vi "Main.vi"(11 "Module Admin":refnum<class "Delacor_lib_QMH_Cloneable Module Admin.lvclass">) -> ()   [LabVIEW 2025, in "USB IO.lvlib"]
doc: "This template is based off of the Queued Message Handler design pattern and the Queued Message Handler project template that ships with LabVIEW.\n\nThe main difference is that the queue is private to this module and communication between modules is performed via Broadcast and Request events.\n\nRequest events are wrapped in public API methods and are handled in the Event Handling Loop (EHL) of this VI. Any module can register for Broadcast events sent by this module. The EHL generates messages based on user interface actions.\n\nThe Message Handling Loop (MHL) processes messages generated by the EHL, or by other messages. The messages are string values, so new messages can be added easily to the Message Cases case structure in the MHL. Each message cluster can also provide an optional value for Message Data, which is a variant that can be converted to whatever message-specific data is required.\n_____\nBased on DQMH Dev Tools: Project Template 7.1.2.1547."
uses:
  USB IO.lvlib
  <vilib>/Delacor/Delacor QMH/Libraries/Message Queue_class/Delacor_lib_QMH_Message Queue.lvclass
  Module Data--cluster.ctl
  <vilib>/Utility/miscctls.llb/LVPointTypeDef.ctl
  <vilib>/Delacor/Delacor QMH/Libraries/Message Queue_class/Delacor_lib_QMH_Enqueue Message (Single).vi
  Stop Argument--cluster.ctl
  <vilib>/Delacor/Delacor QMH/Libraries/Cloneable Module Admin_class/Delacor_lib_QMH_Cloneable Module Admin.lvclass
  Display Lines (Reply Payload)--cluster.ctl
  Display Lines Argument--cluster.ctl
  Classes/USB IO generic/USB IO.lvclass
  select child (Reply Payload)--cluster.ctl
  Classes/Hardware Selection.ctl
  select child Argument--cluster.ctl
  Classes/Arduino Uno/Arduino Uno.lvclass
  Classes/USB-6000/USB-6000.lvclass
  read config (Reply Payload)--cluster.ctl
  read config Argument--cluster.ctl
  init device (Reply Payload)--cluster.ctl
  init device Argument--cluster.ctl
  stop device (Reply Payload)--cluster.ctl
  stop device Argument--cluster.ctl
  Controls/Numeric Voltage.ctl
  analog read (Reply Payload)--cluster.ctl
  analog read Argument--cluster.ctl
  digital write (Reply Payload)--cluster.ctl
  digital write Argument--cluster.ctl
  C:/Users/Tyson.Grover/Desktop/Repositories/torque-test-station/Libraries/USB IO/Classes/USB IO generic/USB IO.lvclass
  C:/Users/Tyson.Grover/Desktop/Repositories/torque-test-station/Libraries/USB IO/Classes/USB-6000/USB-6000.lvclass
  C:/Users/Tyson.Grover/Desktop/Repositories/torque-test-station/Libraries/USB IO/Classes/Arduino Uno/Arduino Uno.lvclass
panel:
  out "error out":errorcluster
  out "Status":string
  in  "Simulate EHL Error":bool
  in  "Simulate MHL Error":bool
  # "Other processes communicate with this Module via its Public API (wrappers for its Request Events).\n\nThis Module communicates with other processes via its Broadcast Events.\nAny process that wants to receive these messages can register for this module's Broadcast events."
  # "This template is for the DQMH framework. See the block diagram for more information on how to use this template."
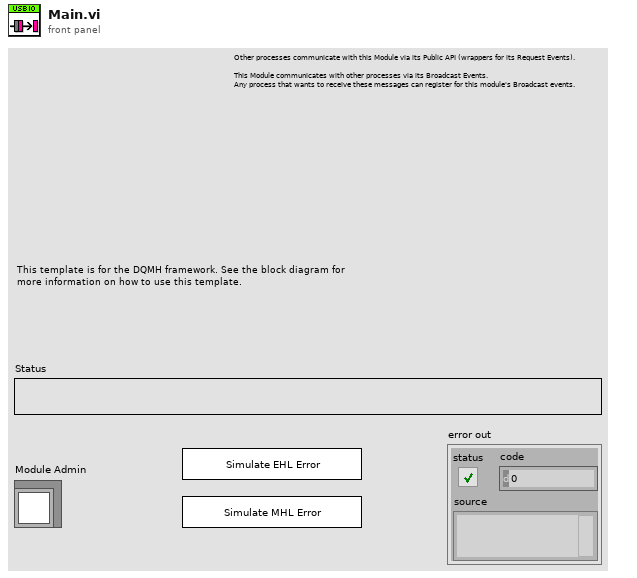
[diagram p1: front panel]
types:
  T1 = typedef "USB IO.lvlib/Request Events--cluster.ctl" = cluster{"Stop Module":refnum<user-event>, "Show Panel":refnum<user-event>, "Hide Panel":refnum<user-event>, "Show Diagram":refnum<user-event>, "Get Module Execution Status":refnum<user-event>, "Display Lines":refnum<user-event>, "select child":refnum<user-event>, "read config":refnum<user-event>, "init":refnum<user-event>, "init device":refnum<user-event>, "stop device":refnum<user-event>, "analog read":refnum<user-event>, "digital write":refnum<user-event>}
  T2 = typedef "USB IO.lvlib/Module Data--cluster.ctl" = cluster{"Status":string, "USB IO.lvlib:USB IO.lvclass":refnum<class "USB IO.lvclass">}
  T3 = enum32{"invalid lock state", "Not Locked", "Locked (No Password)", "Password-protected"}
  T4 = typedef "USB IO.lvlib/Stop Argument--cluster.ctl" = cluster{"Module ID":i32, "Origin":string, "Exit via Stop Module Req?":bool, "Wait for Module to stop?":bool}
  T5 = typedef "USB IO.lvlib/Display Lines Argument--cluster.ctl" = cluster{"Module ID":i32, "Wait Notifier":refnum<notifier>, "wait for reply":bool}
  T6 = typedef "USB IO.lvlib/select child Argument--cluster.ctl" = cluster{"Module ID":i32, "Hardware":T7, "Wait Notifier":refnum<notifier>, "wait for reply":bool}
  T7 = typedef "Hardware Selection.ctl" = enum16{"Simulation", "USB-6000", "USB-6001", "Arduino Uno"}
  T8 = typedef "USB IO.lvlib/read config Argument--cluster.ctl" = cluster{"Module ID":i32, "Path":path, "Wait Notifier":refnum<notifier>, "wait for reply":bool}
  T9 = typedef "USB IO.lvlib/init device Argument--cluster.ctl" = cluster{"Module ID":i32, "Variant":variant, "Wait Notifier":refnum<notifier>, "wait for reply":bool}
  T10 = typedef "USB IO.lvlib/stop device Argument--cluster.ctl" = cluster{"Module ID":i32, "Wait Notifier":refnum<notifier>, "wait for reply":bool}
  T11 = typedef "USB IO.lvlib/analog read Argument--cluster.ctl" = cluster{"Module ID":i32, "Line":string, "Wait Notifier":refnum<notifier>, "wait for reply":bool}
  T12 = typedef "USB IO.lvlib/digital write Argument--cluster.ctl" = cluster{"Module ID":i32, "Line":string, "On/Off":bool, "Wait Notifier":refnum<notifier>, "wait for reply":bool}
  T13 = typedef "LVPointTypeDef.ctl" = cluster{"Horizontal":i16, "Vertical":i16}
  T14 = enum32{"Invalid", "Standard", "Closed", "Hidden", "Minimized", "Maximized"}
  T15 = typedef "USB IO.lvlib/Display Lines (Reply Payload)--cluster.ctl" = cluster{"Module ID":i32, "Lines":string[], "Values":i32[], "error":errorcluster}
  T16 = typedef "USB IO.lvlib/select child (Reply Payload)--cluster.ctl" = cluster{"Module ID":i32, "error":errorcluster}
  T17 = typedef "USB IO.lvlib/read config (Reply Payload)--cluster.ctl" = cluster{"Module ID":i32, "error":errorcluster}
  T18 = typedef "USB IO.lvlib/init device (Reply Payload)--cluster.ctl" = cluster{"Module ID":i32, "error":errorcluster}
  T19 = typedef "USB IO.lvlib/stop device (Reply Payload)--cluster.ctl" = cluster{"Module ID":i32, "error":errorcluster}
  T20 = typedef "USB IO.lvlib/analog read (Reply Payload)--cluster.ctl" = cluster{"Module ID":i32, "Voltage":T21, "error":errorcluster}
  T21 = typedef "Numeric Voltage.ctl" = dbl
  T22 = typedef "USB IO.lvlib/digital write (Reply Payload)--cluster.ctl" = cluster{"Module ID":i32, "error":errorcluster}
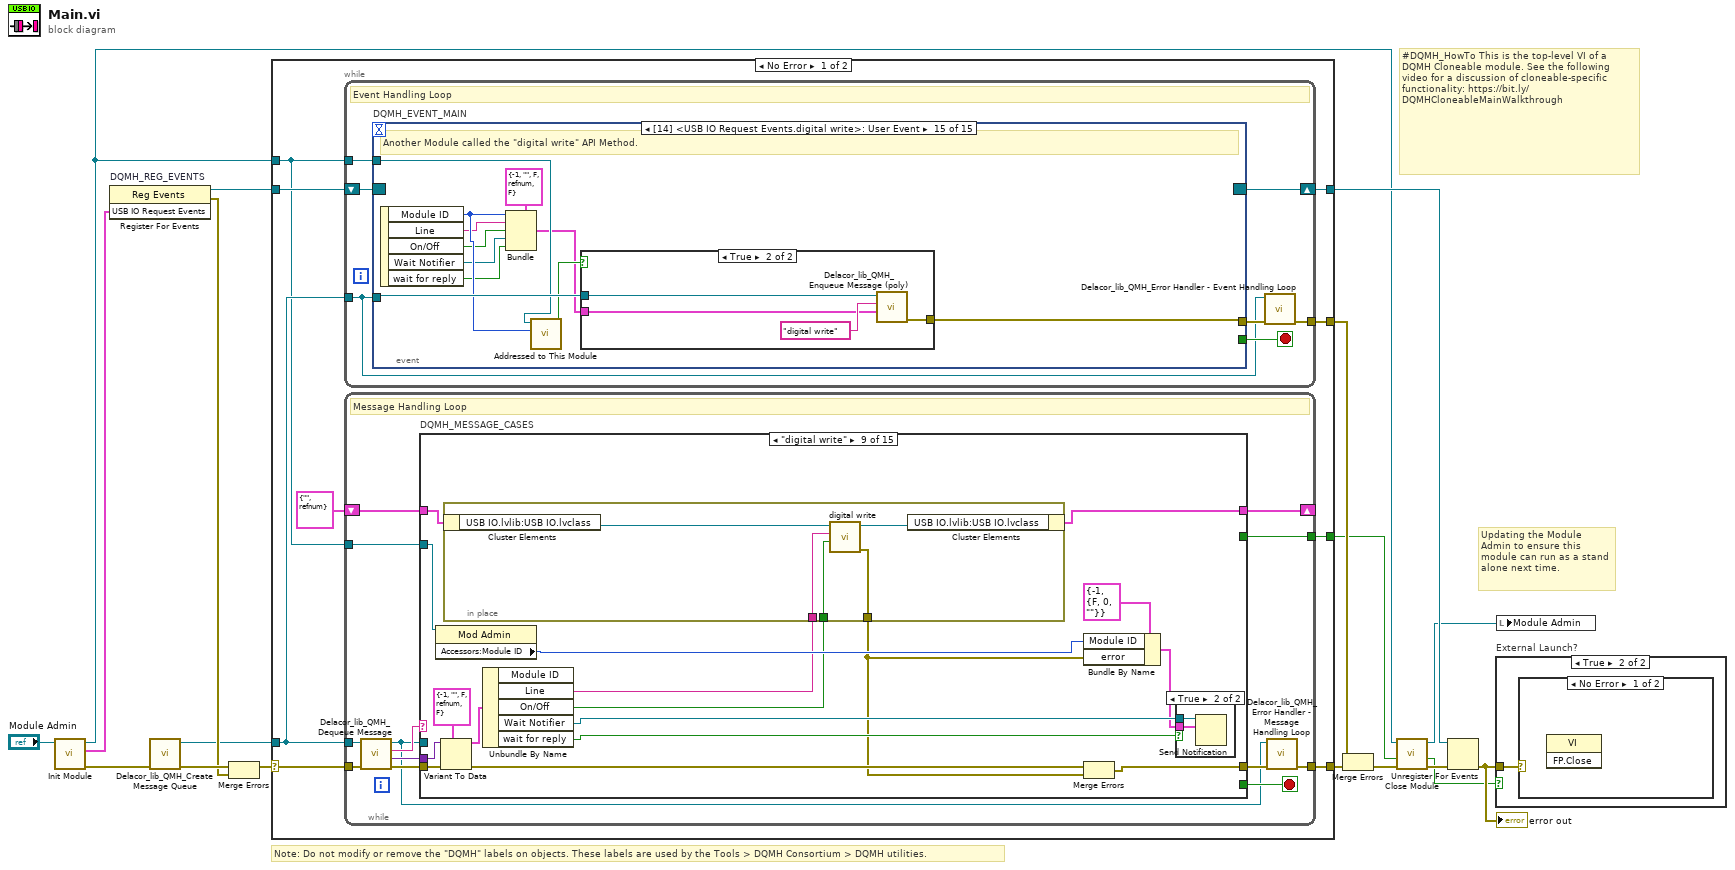
[diagram p0: block diagram]
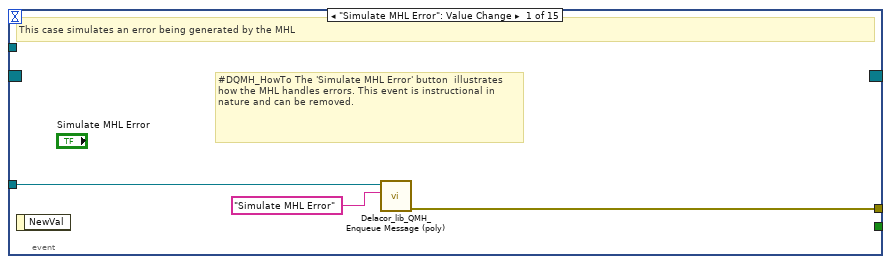
[diagram p2: hidden frame]
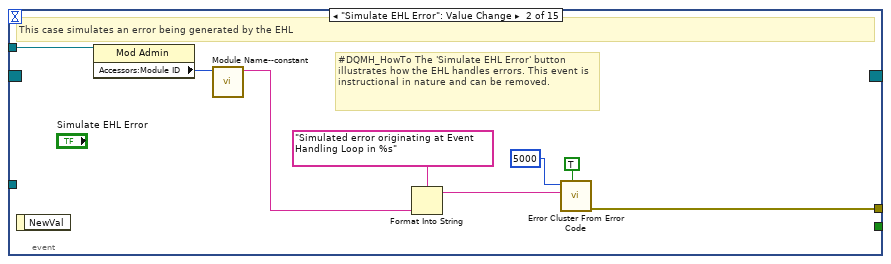
[diagram p3: hidden frame]
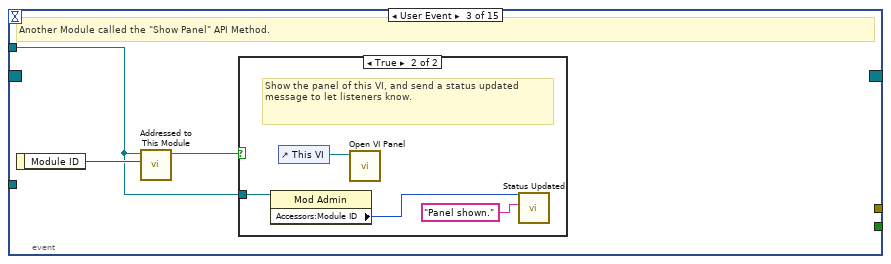
[diagram p4: hidden frame]
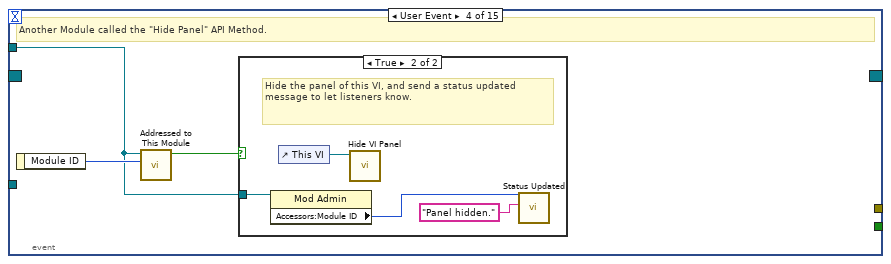
[diagram p6: hidden frame]
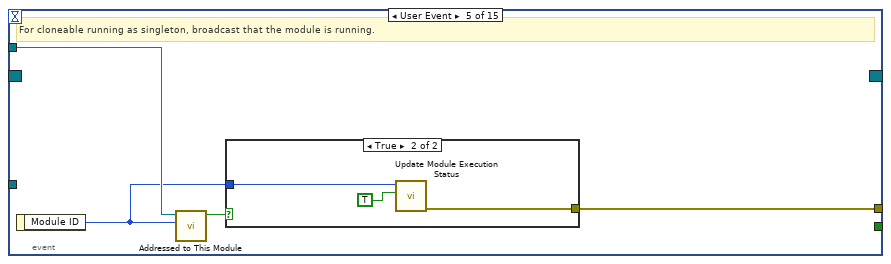
[diagram p8: hidden frame]
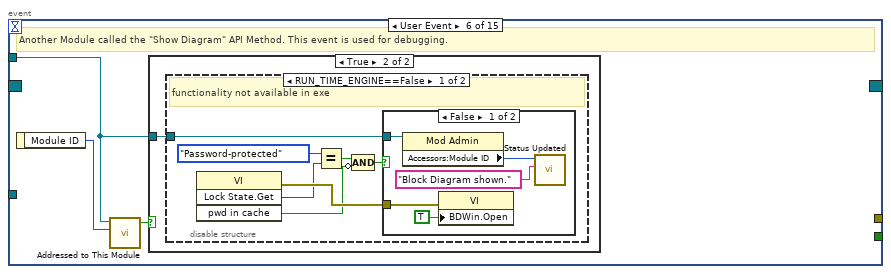
[diagram p10: hidden frame]
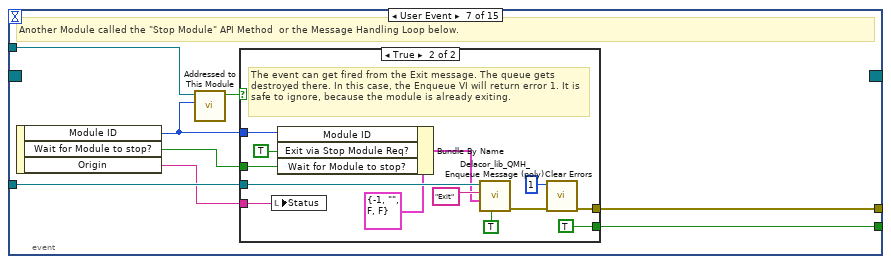
[diagram p14: hidden frame]
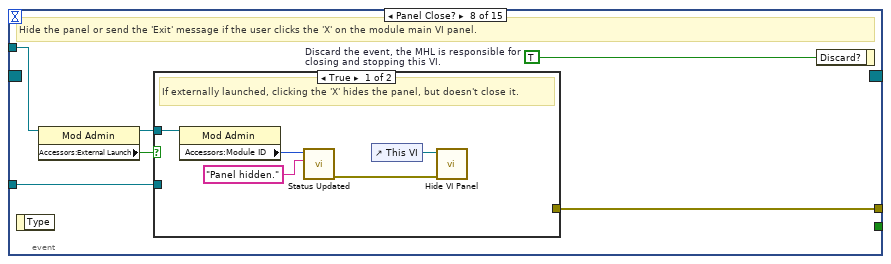
[diagram p16: hidden frame]
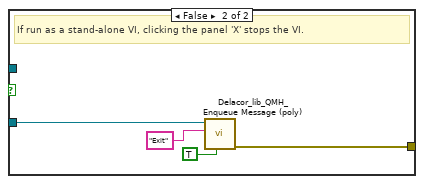
[diagram p17: hidden frame]
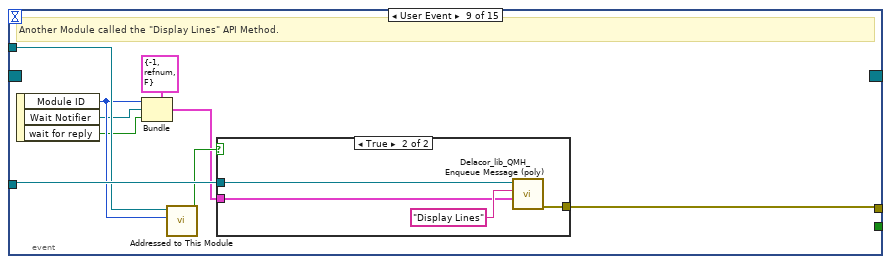
[diagram p18: hidden frame]
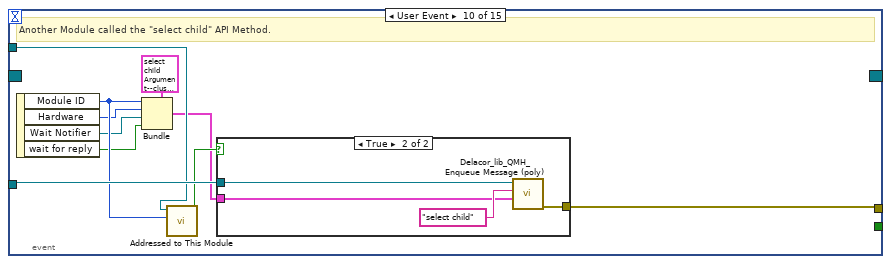
[diagram p20: hidden frame]
diagram:
  # "#DQMH_HowTo This is the top-level VI of a DQMH Cloneable module. See the following video for a discussion of cloneable-specific functionality: https://bit.ly/DQMHCloneableMainWalkthrough"
  # "Note: Do not modify or remove the \"DQMH\" labels on objects. These labels are used by the Tools > DQMH Consortium > DQMH utilities."
  # "Updating the Module Admin to ensure this module can run as a stand alone next time."
  n1 = call "Init Module.vi"("Cloneable Module Admin in"="Module Admin") -> ("error out"=w15:errorcluster, "USB IO Request Events"=w7:T1, "Cloneable Module Admin out"=w4:refnum<class "Delacor_lib_QMH_Cloneable Module Admin.lvclass">)  [unwired: 8 in]
  n2 = register-events "DQMH_REG_EVENTS"(w7) -> (reference out=w8:refnum<event-registration>, error out=w10:errorcluster)  [unwired: 2 in]
  n3 = call <vilib>:"Delacor_lib_QMH_Create Message Queue.vi"("error in"=w15) -> ("error out"=w12:errorcluster, "Message Queue"=w6:refnum<class "Delacor_lib_QMH_Message Queue.lvclass">)  [unwired: 9 in]
  n4 = Merge Errors(w12, w10) -> (w11:errorcluster)
  n5 = case shown="No Error" w11 {
    selector: w11 -> [w25 w482]
    tunnel: [w27 w481] -> w16
    tunnel: [w24 w480] -> w9
    tunnel: w8 -> [w22 w480]
    tunnel: w6 -> [w21 w473]
    tunnel: [w26 _] -> w17
    tunnel: w4 -> [w20 w476]
    tunnel: [w19 _] -> w2
    frame No Error {
      n6 = while {
        tunnel: w21 -> [w28]
        shift-right: [w31] -> w24
        shift-left: w22 -> [w32]
        tunnel: [w33] -> w26
        tunnel: w20 -> [w29]
        stop <- w30 stop-if-true
        # "Event Handling Loop"
        n7 = event "DQMH_EVENT_MAIN" shown="[14] <USB IO Request Events.digital write>: User Event" {
          selector: w32 -> [_ _ _ _ _ _ _ _ _ _ _ _ _ _ _]
          dyn-events: [_ _ _ _ _ _ _ _ _ _ _ _ _ _ _] -> w31
          timeout: _ -> [_ _ _ _ _ _ _ _ _ _ _ _ _ _ _]
          tunnel: [_ _ _ _ _ _ w86 _ _ _ _ _ _ _ _] -> w30
          tunnel: w28 -> [w36 _ _ _ _ _ w89 w106 w127 w141 w155 w169 w182 w196 w211]
          tunnel: [w37 w45 _ _ w63 _ w90 w109 w119 w132 w146 w160 w174 w187 w201] -> w34
          tunnel: w29 -> [_ w44 w46 w53 w61 w67 w88 w107 w125 w139 w153 w167 w180 w194 w209]
          event "Simulate MHL Error": Value Change {
            # "#DQMH_HowTo The 'Simulate MHL Error' button  illustrates how the MHL handles errors. This event is instructional in nature and can be removed."
            # "This case simulates an error being generated by the MHL"
            n8 = event-data() -> ()  [unwired: 1 in, 1 out]
            n9 = call-poly <vilib>:"Delacor_lib_QMH_Enqueue Message (poly).vi"("Message"="Simulate MHL Error", "Message Queue in"=w36) -> ("error out"=w37:errorcluster)  [unwired: 8 in, 1 out]
          }
          event "Simulate EHL Error": Value Change {
            # "#DQMH_HowTo The 'Simulate EHL Error' button  illustrates how the EHL handles errors. This event is instructional in nature and can be removed."
            # "This case simulates an error being generated by the EHL"
            n10 = event-data() -> ()  [unwired: 1 in, 1 out]
            n11 = property on="Property Node" class="Mod Admin"(reference=w44) -> ("Accessors:Module ID"=w43:i32)  [unwired: 1 in, 2 out]
            n12 = call "Module Name--constant.vi"("Module ID"=w43) -> ("Module Name"=w38:string)  [unwired: 10 in]
            n13 = Format Into String(format string="Simulated error originating at Event Handling Loop in %s", w38) -> (resulting string=w41:string)  [unwired: 2 in, 1 out]
            n14 = call <vilib>:"Error Cluster From Error Code.vi"("show call chain? (False)"=TRUE, "error message (\"\")"=w41, "error code (0)"=5000) -> ("error out"=w45:errorcluster)  [unwired: 6 in]
          }
          event User Event {
            # "Another Module called the \"Show Panel\" API Method."
            n15 = event-data() -> ("Module ID"=w47:i32)  [unwired: 1 in]
            n16 = call "Addressed to This Module.vi"("Module ID from Argument"=w47, "Module Admin"=w46) -> ("Addressed to this instance?"=w48:bool)  [unwired: 8 in, 1 out]
            n17 = case shown="True" w48 {
              tunnel: w46 -> [_ w50]
              frame False {
              }
              frame True {
                # "Show the panel of this VI, and send a status updated message to let listeners know."
                n18 = property on="Property Node" class="Mod Admin"(reference=w50) -> ("Accessors:Module ID"=w49:i32)  [unwired: 1 in, 2 out]
                n19 = control-ref of="This VI"() -> (w52:refnum<vi>)
                n20 = call "Open VI Panel.vi"("VI"=w52) -> ()  [unwired: 10 in, 1 out]
                n21 = call "Status Updated.vi"("Status"="Panel shown." ("format string"), "Module ID"=w49) -> ()  [unwired: 9 in, 1 out]
              }
            }
          }
          event User Event {
            # "Another Module called the \"Hide Panel\" API Method."
            n22 = event-data() -> ("Module ID"=w54:i32)  [unwired: 1 in]
            n23 = call "Addressed to This Module.vi"("Module ID from Argument"=w54, "Module Admin"=w53) -> ("Addressed to this instance?"=w55:bool)  [unwired: 8 in, 1 out]
            n24 = case shown="True" w55 {
              tunnel: w53 -> [_ w57]
              frame False {
              }
              frame True {
                # "Hide the panel of this VI, and send a status updated message to let listeners know."
                n25 = property on="Property Node" class="Mod Admin"(reference=w57) -> ("Accessors:Module ID"=w56:i32)  [unwired: 1 in, 2 out]
                n26 = control-ref of="This VI"() -> (w59:refnum<vi>)
                n27 = call "Hide VI Panel.vi"("VI"=w59) -> ()  [unwired: 10 in, 1 out]
                n28 = call "Status Updated.vi"("Status"="Panel hidden." ("format string"), "Module ID"=w56) -> ()  [unwired: 9 in, 1 out]
              }
            }
          }
          event User Event {
            # "For cloneable running as singleton, broadcast that the module is running."
            n29 = event-data() -> ("Module ID"=w60:i32)  [unwired: 1 in]
            n30 = call "Addressed to This Module.vi"("Module ID from Argument"=w60, "Module Admin"=w61) -> ("Addressed to this instance?"=w62:bool)  [unwired: 8 in, 1 out]
            n31 = case shown="True" w62 {
              tunnel: [_ w66] -> w63
              tunnel: w60 -> [_ w65]
              frame False {
              }
              frame True {
                n32 = call "Update Module Execution Status.vi"("Running?"=TRUE, "Module ID"=w65) -> ("error out"=w66:errorcluster)  [unwired: 9 in]
              }
            }
          }
          event User Event {
            # "Another Module called the \"Show Diagram\" API Method. This event is used for debugging."
            n33 = event-data() -> ("Module ID"=w68:i32)  [unwired: 1 in]
            n34 = call "Addressed to This Module.vi"("Module ID from Argument"=w68, "Module Admin"=w67) -> ("Addressed to this instance?"=w69:bool)  [unwired: 8 in, 1 out]
            n35 = case shown="True" w69 {
              tunnel: w67 -> [_ w70]
              frame False {
              }
              frame True {
                n36 = disable-structure shown="RUN_TIME_ENGINE==False" {
                  disable-tunnel: w70 -> [w71 _]
                  frame condition #0 (active) {
                    # "functionality not available in exe"
                    n37 = invoke on="Invoke Node" class="VI" method="Lock State.Get"() -> (error out=w77:errorcluster, "Get Lock State"=w76:T3, "pwd in cache"=w73:bool)  [unwired: 4 in, 1 out]
                    n38 = Equal?(x=T3."Password-protected", y=w76) -> (x = y?=w74:bool)
                    n39 = Compound Arithmetic op=AND(w74, invert w73) -> (w72:bool)
                    n40 = case shown="False" w72 {
                      tunnel: w77 -> [w82 _]
                      tunnel: w71 -> [w79 _]
                      frame False {
                        n41 = property on="Property Node" class="Mod Admin"(reference=w79) -> ("Accessors:Module ID"=w78:i32)  [unwired: 1 in, 2 out]
                        n42 = property on="Property Node" class="VI"(error in=w82, "BDWin.Open"=TRUE ("Block Diagram Window:Open")) -> ()  [unwired: 1 in, 2 out]
                        n43 = call "Status Updated.vi"("Status"="Block Diagram shown." ("format string"), "Module ID"=w78) -> ()  [unwired: 9 in, 1 out]
                      }
                      frame True {
                        # "Password-protected VI, and the password is not in the cache. Do not show the diagram."
                      }
                    }
                  }
                  frame condition #1 {
                  }
                }
              }
            }
          }
          event User Event {
            # "Another Module called the \"Stop Module\" API Method  or the Message Handling Loop below."
            n44 = event-data() -> ("Module ID"=w84:i32, "Wait for Module to stop?"=w85:bool, "Origin"=w83:string)  [unwired: 1 in]
            n45 = call "Addressed to This Module.vi"("Module ID from Argument"=w84, "Module Admin"=w88) -> ("Addressed to this instance?"=w87:bool)  [unwired: 8 in, 1 out]
            n46 = case shown="True" w87 {
              tunnel: [_ w102] -> w90
              tunnel: w89 -> [_ w98]
              tunnel: [_ TRUE] -> w86
              tunnel: w85 -> [_ w93]
              tunnel: w84 -> [_ w95]
              tunnel: w83 -> [_ w91]
              frame False {
              }
              frame True {
                # "The event can get fired from the Exit message. The queue gets destroyed there. In this case, the Enqueue VI will return error 1. It is safe to ignore, because the module is already exiting."
                n47 = local write "Status"(w91) -> ()
                n48 = Bundle By Name(cluster=T4 {"Module ID"=-1, "Origin"="", "Exit via Stop Module Req?"=FALSE, "Wait for Module to stop?"=FALSE} ("Stop Argument"), "Module ID"=w95, "Exit via Stop Module Req?"=TRUE, "Wait for Module to stop?"=w93) -> (w92:T4)
                n49 = call-poly <vilib>:"Delacor_lib_QMH_Enqueue Message (poly).vi"("Priority Message? (F)"=TRUE, "Message Data"=w92, "Message"="Exit", "Message Queue in"=w98) -> ("error out"=w103:errorcluster)  [unwired: 6 in, 1 out]
                n50 = call <vilib>:"Clear Errors.vi"("error in (no error)"=w103, "specific error code to clear (0: all)"=1) -> ("error out"=w102:errorcluster)  [unwired: 4 in, 1 out]
              }
            }
          }
          event Panel Close? {
            w108 = TRUE  # Discard the event, the MHL is responsible for closing and stopping this VI.
            # "Hide the panel or send the 'Exit' message if the user clicks the 'X' on the module main VI panel."
            n51 = event-data() -> ()  [unwired: 1 in, 1 out]
            n52 = property on="Property Node" class="Mod Admin"(reference=w107) -> (reference out=w104:refnum<class "Delacor_lib_QMH_Cloneable Module Admin.lvclass">, "Accessors:External Launch"=w105:bool)  [unwired: 1 in, 1 out]
            n53 = case shown="True" w105 {
              tunnel: w106 -> [_ w117]
              tunnel: [_ w118] -> w109
              tunnel: w104 -> [w112 _]
              frame True {
                # "If externally launched, clicking the 'X' hides the panel, but doesn't close it."
                n54 = property on="Property Node" class="Mod Admin"(reference=w112) -> ("Accessors:Module ID"=w111:i32)  [unwired: 1 in, 2 out]
                n55 = call "Status Updated.vi"("Status"="Panel hidden." ("format string"), "Module ID"=w111) -> ("error out"=w110:errorcluster)  [unwired: 9 in]
                n56 = control-ref of="This VI"() -> (w114:refnum<vi>)
                n57 = call "Hide VI Panel.vi"("error in"=w110, "VI"=w114) -> ()  [unwired: 9 in, 1 out]
              }
              frame False {
                # "If run as a stand-alone VI, clicking the panel 'X' stops the VI."
                n58 = call-poly <vilib>:"Delacor_lib_QMH_Enqueue Message (poly).vi"("Priority Message? (F)"=TRUE, "Message"="Exit", "Message Queue in"=w117) -> ("error out"=w118:errorcluster)  [unwired: 7 in, 1 out]
              }
            }
            n59 = event-data ("Event Filter Node")("Discard?"=w108) -> ()  [unwired: 1 in, 1 out]
          }
          event User Event {
            # "Another Module called the \"Display Lines\" API Method."
            n60 = event-data() -> ("Module ID"=w122:i32, "Wait Notifier"=w121:refnum<notifier>, "wait for reply"=w120:bool)  [unwired: 1 in]
            n61 = Bundle(cluster=T5 {"Module ID"=-1, "Wait Notifier"=refnum, "wait for reply"=FALSE} ("Display Lines Argument"), "Module ID"=w122, "Wait Notifier"=w121, "wait for reply"=w120) -> (w123:T5)
            n62 = call "Addressed to This Module.vi"("Module ID from Argument"=w122, "Module Admin"=w125) -> ("Addressed to this instance?"=w126:bool)  [unwired: 8 in, 1 out]
            n63 = case shown="True" w126 {
              tunnel: w127 -> [_ w131]
              tunnel: w123 -> [_ w129]
              tunnel: [_ w128] -> w119
              frame False {
              }
              frame True {
                n64 = call-poly <vilib>:"Delacor_lib_QMH_Enqueue Message (poly).vi"("Message Data"=w129, "Message"="Display Lines", "Message Queue in"=w131) -> ("error out"=w128:errorcluster)  [unwired: 7 in, 1 out]
              }
            }
          }
          event User Event {
            # "Another Module called the \"select child\" API Method."
            n65 = event-data() -> ("Module ID"=w136:i32, "Hardware"=w135:T7, "Wait Notifier"=w134:refnum<notifier>, "wait for reply"=w133:bool)  [unwired: 1 in]
            n66 = Bundle(cluster=T6 {"Module ID"=-1, "Hardware"=enum."USB-6000", "Wait Notifier"=refnum, "wait for reply"=FALSE} ("select child Argument"), "Module ID"=w136, "Hardware"=w135, "Wait Notifier"=w134, "wait for reply"=w133) -> (w137:T6)
            n67 = call "Addressed to This Module.vi"("Module ID from Argument"=w136, "Module Admin"=w139) -> ("Addressed to this instance?"=w140:bool)  [unwired: 8 in, 1 out]
            n68 = case shown="True" w140 {
              tunnel: w141 -> [_ w145]
              tunnel: w137 -> [_ w143]
              tunnel: [_ w142] -> w132
              frame False {
              }
              frame True {
                n69 = call-poly <vilib>:"Delacor_lib_QMH_Enqueue Message (poly).vi"("Message Data"=w143, "Message"="select child", "Message Queue in"=w145) -> ("error out"=w142:errorcluster)  [unwired: 7 in, 1 out]
              }
            }
          }
          event User Event {
            # "Another Module called the \"read config\" API Method."
            n70 = event-data() -> ("Module ID"=w150:i32, "Path"=w149:path, "Wait Notifier"=w148:refnum<notifier>, "wait for reply"=w147:bool)  [unwired: 1 in]
            n71 = Bundle(cluster=T8 {"Module ID"=-1, "Path"=path "", "Wait Notifier"=refnum, "wait for reply"=FALSE} ("read config Argument"), "Module ID"=w150, "Path"=w149, "Wait Notifier"=w148, "wait for reply"=w147) -> (w151:T8)
            n72 = call "Addressed to This Module.vi"("Module ID from Argument"=w150, "Module Admin"=w153) -> ("Addressed to this instance?"=w154:bool)  [unwired: 8 in, 1 out]
            n73 = case shown="True" w154 {
              tunnel: w155 -> [_ w159]
              tunnel: w151 -> [_ w157]
              tunnel: [_ w156] -> w146
              frame False {
              }
              frame True {
                n74 = call-poly <vilib>:"Delacor_lib_QMH_Enqueue Message (poly).vi"("Message Data"=w157, "Message"="read config", "Message Queue in"=w159) -> ("error out"=w156:errorcluster)  [unwired: 7 in, 1 out]
              }
            }
          }
          event User Event {
            # "Another Module called the \"init device\" API Method."
            n75 = event-data() -> ("Module ID"=w164:i32, "Variant"=w163:variant, "Wait Notifier"=w162:refnum<notifier>, "wait for reply"=w161:bool)  [unwired: 1 in]
            n76 = Bundle(cluster=T9 {"Module ID"=-1, "Variant"=variant, "Wait Notifier"=refnum, "wait for reply"=FALSE} ("init device Argument"), "Module ID"=w164, "Variant"=w163, "Wait Notifier"=w162, "wait for reply"=w161) -> (w165:T9)
            n77 = call "Addressed to This Module.vi"("Module ID from Argument"=w164, "Module Admin"=w167) -> ("Addressed to this instance?"=w168:bool)  [unwired: 8 in, 1 out]
            n78 = case shown="True" w168 {
              tunnel: w169 -> [_ w173]
              tunnel: w165 -> [_ w171]
              tunnel: [_ w170] -> w160
              frame False {
              }
              frame True {
                n79 = call-poly <vilib>:"Delacor_lib_QMH_Enqueue Message (poly).vi"("Message Data"=w171, "Message"="init device", "Message Queue in"=w173) -> ("error out"=w170:errorcluster)  [unwired: 7 in, 1 out]
              }
            }
          }
          event User Event {
            # "Another Module called the \"stop device\" API Method."
            n80 = event-data() -> ("Module ID"=w177:i32, "Wait Notifier"=w176:refnum<notifier>, "wait for reply"=w175:bool)  [unwired: 1 in]
            n81 = Bundle(cluster=T10 {"Module ID"=-1, "Wait Notifier"=refnum, "wait for reply"=FALSE} ("stop device Argument"), "Module ID"=w177, "Wait Notifier"=w176, "wait for reply"=w175) -> (w178:T10)
            n82 = call "Addressed to This Module.vi"("Module ID from Argument"=w177, "Module Admin"=w180) -> ("Addressed to this instance?"=w181:bool)  [unwired: 8 in, 1 out]
            n83 = case shown="True" w181 {
              tunnel: w182 -> [_ w186]
              tunnel: w178 -> [_ w184]
              tunnel: [_ w183] -> w174
              frame False {
              }
              frame True {
                n84 = call-poly <vilib>:"Delacor_lib_QMH_Enqueue Message (poly).vi"("Message Data"=w184, "Message"="stop device", "Message Queue in"=w186) -> ("error out"=w183:errorcluster)  [unwired: 7 in, 1 out]
              }
            }
          }
          event User Event {
            # "Another Module called the \"analog read\" API Method."
            n85 = event-data() -> ("Module ID"=w191:i32, "Line"=w190:string, "Wait Notifier"=w189:refnum<notifier>, "wait for reply"=w188:bool)  [unwired: 1 in]
            n86 = Bundle(cluster=T11 {"Module ID"=-1, "Line"="", "Wait Notifier"=refnum, "wait for reply"=FALSE} ("analog read Argument"), "Module ID"=w191, "Line"=w190, "Wait Notifier"=w189, "wait for reply"=w188) -> (w192:T11)
            n87 = call "Addressed to This Module.vi"("Module ID from Argument"=w191, "Module Admin"=w194) -> ("Addressed to this instance?"=w195:bool)  [unwired: 8 in, 1 out]
            n88 = case shown="True" w195 {
              tunnel: w196 -> [_ w200]
              tunnel: w192 -> [_ w198]
              tunnel: [_ w197] -> w187
              frame False {
              }
              frame True {
                n89 = call-poly <vilib>:"Delacor_lib_QMH_Enqueue Message (poly).vi"("Message Data"=w198, "Message"="analog read", "Message Queue in"=w200) -> ("error out"=w197:errorcluster)  [unwired: 7 in, 1 out]
              }
            }
          }
          event User Event {
            # "Another Module called the \"digital write\" API Method."
            n90 = event-data() -> ("Module ID"=w206:i32, "Line"=w205:string, "On/Off"=w204:bool, "Wait Notifier"=w203:refnum<notifier>, "wait for reply"=w202:bool)  [unwired: 1 in]
            n91 = Bundle(cluster=T12 {"Module ID"=-1, "Line"="", "On/Off"=FALSE, "Wait Notifier"=refnum, "wait for reply"=FALSE} ("digital write Argument"), "Module ID"=w206, "Line"=w205, "On/Off"=w204, "Wait Notifier"=w203, "wait for reply"=w202) -> (w207:T12)
            n92 = call "Addressed to This Module.vi"("Module ID from Argument"=w206, "Module Admin"=w209) -> ("Addressed to this instance?"=w210:bool)  [unwired: 8 in, 1 out]
            n93 = case shown="True" w210 {
              tunnel: w211 -> [_ w215]
              tunnel: w207 -> [_ w213]
              tunnel: [_ w212] -> w201
              frame False {
              }
              frame True {
                n94 = call-poly <vilib>:"Delacor_lib_QMH_Enqueue Message (poly).vi"("Message Data"=w213, "Message"="digital write", "Message Queue in"=w215) -> ("error out"=w212:errorcluster)  [unwired: 7 in, 1 out]
              }
            }
          }
        }
        n95 = call-dynamic "Delacor_lib_QMH_Error Handler - Event Handling Loop.vi"("error in"=w34, "Message Queue in"=w28) -> ("dup error in"=w33:errorcluster)  [unwired: 8 in, 1 out]
      }
      n96 = while {
        tunnel: w21 -> [w216]
        shift-right: [w223] -> _
        shift-left: T2 {"Status"="", "USB IO.lvlib:USB IO.lvclass"=refnum} ("Data Cluster") -> [w224]
        tunnel: w25 -> [w227]
        tunnel: [w225] -> w27
        tunnel: w20 -> [w218]
        tunnel: [w217] -> w19
        stop <- w222 stop-if-true
        # "Message Handling Loop"
        n97 = call-dynamic "Delacor_lib_QMH_Dequeue Message.vi"("error in"=w227, "Message Queue in"=w216) -> ("error out"=w226:errorcluster, "Message Data"=w220:variant, "Message"=w221:string, "Message Queue out"=w219:refnum<class "Delacor_lib_QMH_Message Queue.lvclass">)  [unwired: 6 in]
        n98 = case "DQMH_MESSAGE_CASES" shown="\"digital write\"" w221 {
          selector: w221 -> [_ _ _ _ _ _ _ _ _ _ _ _ _ _ w462]
          tunnel: w219 -> [_ _ _ _ _ _ _ _ _ _ _ w417 _ w454 _]
          tunnel: w226 -> [w247 w251 w268 w291 w313 w335 w356 w378 w402 w412 w414 w426 w443 w460 w471]
          tunnel: [w245 w251 w259 w282 w304 w326 w347 w369 w393 w411 w414 w422 w442 w455 w472] -> w228
          tunnel: w224 -> [w238 w250 w255 w279 w301 w323 w344 w366 w390 w410 w413 w421 w440 w453 w469]
          tunnel: [w237 w250 w256 w277 w300 w322 w343 w365 w389 w410 w413 w421 w440 w453 w469] -> w223
          tunnel: [_ _ _ _ _ _ _ _ _ _ _ _ _ w452 _] -> w222
          tunnel: w220 -> [_ _ w266 w289 w311 w333 w354 w376 w400 _ _ w420 _ w450 _]
          tunnel: w218 -> [w233 _ w257 w280 w302 w324 w345 w367 w391 _ _ w419 w438 w445 w468]
          tunnel: [_ _ _ _ _ _ _ _ _ _ _ _ _ w448 _] -> w217
          frame "Initialize" {
            w230 = "Initial Message" ("Initial Message")
            # "#DQMH_CodeNeeded - Initialize the appearance of the front panel."
            # "#DQMH_CodeNeeded - Initialize your state data here."
            # "Initialize - Any operation that needs to be done before the module can receive messages. Synchronize Caller Events.vi will inform Start Module.vi that the module has launched and is ready to receive messages. Module Did Init.vi will broadcast that the module initialized."
            n99 = call "Synchronize Caller Events.vi"("error in"=w247, "Module Admin"=w233) -> ("error out"=w246:errorcluster, "Module Admin out"=w232:refnum<class "Delacor_lib_QMH_Cloneable Module Admin.lvclass">)  [unwired: 8 in]
            n100 = property on="Property Node" class="Mod Admin"(reference=w232) -> ("Accessors:Module ID"=w229:i32, "Accessors:External Launch"=w234:bool)  [unwired: 1 in, 2 out]
            n101 = call "Module Name--constant.vi"("Module ID"=w229) -> ("Module Name"=w242:string)  [unwired: 10 in]
            n102 = property on="Property Node" class="VI"("Front Panel.Title"=w242) -> (reference out=w244:refnum<vi>, error out=w249:errorcluster)  [unwired: 2 in]
            n103 = Select(t=T14."Hidden" ("State"), s=w234, f=T14."Standard" ("State")) -> (s? t:f=w239:T14)
            n104 = invoke on="Invoke Node" class="VI" method="FP.Open"(reference=w244, error in=w249, "State"=w239) -> (reference out=w243:refnum<vi>, error out=w248:errorcluster)  [unwired: 2 in, 3 out]
            n105 = Bundle By Name(cluster=w238, "Status"=w230) -> (w237:T2)
            n106 = invoke on="Invoke Node" class="VI" method="FP.Center"(reference=w243, error in=w248) -> ()  [unwired: 1 in, 3 out]
            n107 = property on="Pane" class="Pane"("Origin"=T13 {"Horizontal"=0, "Vertical"=0}) -> ()  [unwired: 2 in, 2 out]
            n108 = call "Module Name--constant.vi"("Module ID"=w229) -> ("Module Name"=w235:string)  [unwired: 10 in]
            n109 = call "Module Did Init.vi"("error in"=w246, "Initialized?"=TRUE, "Origin"=w235, "Module ID"=w229) -> ("error out"=w245:errorcluster)  [unwired: 7 in]
            "Status" <- w230
          }
          frame "---Module Specific---" {
            # "Separator -- The following cases handle messages specific to this Module."
          }
          frame "Display Lines" {
            n110 = property class="Mod Admin"(reference=w257) -> ("Accessors:Module ID"=w258:i32)  [unwired: 1 in, 2 out]
            n111 = Variant To Data(error in=w268, type=T5 {"Module ID"=-1, "Wait Notifier"=refnum, "wait for reply"=FALSE} ("Display Lines Argument"), Variant=w266) -> (data=w264:T5, error out=w267:errorcluster)
            n112 = in-place {
              in-place-border: [w271] -> w254
              in-place-border: [w270] -> w253
              in-place-border: [w269] -> w252
              n113 = in-place-cluster #1(w255) -> ("USB IO.lvlib:USB IO.lvclass"=w273:refnum<class "USB IO.lvclass">)
              n114 = call-dynamic "display lines.vi"("USB IO in"=w273) -> ("error out"=w269:errorcluster, "Values"=w270:i32[], "Lines"=w271:string[], "USB IO out"=w272:refnum<class "USB IO.lvclass">)  [unwired: 7 in]
              n115 = in-place-cluster #1("USB IO.lvlib:USB IO.lvclass"=w272) -> (w256:T2)
            }
            n116 = Unbundle By Name(w264) -> ("Wait Notifier"=w263:refnum<notifier>, "wait for reply"=w262:bool)  [unwired: 1 out]
            n117 = Bundle By Name(cluster=T15 {"Module ID"=-1, "Lines"=[], "Values"=[], "error"={"status"=FALSE, "code"=0, "source"=""}} ("Display Lines (Reply Payload)"), "Module ID"=w258, "Lines"=w254, "Values"=w253, "error"=w252) -> (w261:T15)
            n118 = Merge Errors(w267, w252) -> (w259:errorcluster)
            n119 = case "DQMH_FIRE_NOTIFIER" shown="True" w262 {
              tunnel: w263 -> [_ w275]
              tunnel: w261 -> [_ w274]
              frame False {
              }
              frame True {
                n120 = Send Notification(notification=w274, notifier=w275) -> ()  [unwired: 1 in, 2 out]
              }
            }
          }
          frame "select child" {
            w276 = errorcluster {"status"=FALSE, "code"=0, "source"=""} ("error")
            n121 = property class="Mod Admin"(reference=w280) -> ("Accessors:Module ID"=w281:i32)  [unwired: 1 in, 2 out]
            n122 = Variant To Data(error in=w291, type=T6 {"Module ID"=-1, "Hardware"=enum."USB-6000", "Wait Notifier"=refnum, "wait for reply"=FALSE} ("select child Argument"), Variant=w289) -> (data=w287:T6, error out=w290:errorcluster)
            n123 = Unbundle By Name(w287) -> ("Hardware"=w278:T7, "Wait Notifier"=w286:refnum<notifier>, "wait for reply"=w285:bool)  [unwired: 1 out]
            n124 = in-place {
              in-place-border: w278 -> [w293]
              n125 = in-place-cluster #2(w279) -> ()  [unwired: 1 out]
              n126 = case shown="\"USB-6000\", Default" w293 {
                tunnel: [refnum<class "USB-6000.lvclass"> refnum ("USB IO.lvlib:USB-6000.lvclass") refnum<class "Arduino Uno.lvclass"> refnum ("USB IO.lvlib:Arduino Uno.lvclass")] -> w292
                frame "USB-6000", Default {
                }
                frame "Arduino Uno" {
                }
              }
              n127 = in-place-cluster #2("USB IO.lvlib:USB IO.lvclass"=w292) -> (w277:T2)
            }
            n128 = Bundle By Name(cluster=T16 {"Module ID"=-1, "error"={"status"=FALSE, "code"=0, "source"=""}} ("select child (Reply Payload)"), "Module ID"=w281, "error"=w276) -> (w284:T16)
            n129 = Merge Errors(w290, w276) -> (w282:errorcluster)
            n130 = case "DQMH_FIRE_NOTIFIER" shown="True" w285 {
              tunnel: w286 -> [_ w297]
              tunnel: w284 -> [_ w296]
              frame False {
              }
              frame True {
                n131 = Send Notification(notification=w296, notifier=w297) -> ()  [unwired: 1 in, 2 out]
              }
            }
          }
          frame "read config" {
            n132 = property class="Mod Admin"(reference=w302) -> ("Accessors:Module ID"=w303:i32)  [unwired: 1 in, 2 out]
            n133 = Variant To Data(error in=w313, type=T8 {"Module ID"=-1, "Path"=path "", "Wait Notifier"=refnum, "wait for reply"=FALSE} ("read config Argument"), Variant=w311) -> (data=w309:T8, error out=w312:errorcluster)
            n134 = Unbundle By Name(w309) -> ("Path"=w299:path, "Wait Notifier"=w308:refnum<notifier>, "wait for reply"=w307:bool)  [unwired: 1 out]
            n135 = in-place {
              in-place-border: w299 -> [w315]
              in-place-border: [w314] -> w298
              n136 = in-place-cluster #3(w301) -> ("USB IO.lvlib:USB IO.lvclass"=w317:refnum<class "USB IO.lvclass">)
              n137 = call-dynamic "read config.vi"("Path"=w315, "USB IO in"=w317) -> ("error out"=w314:errorcluster, "USB IO out"=w316:refnum<class "USB IO.lvclass">)  [unwired: 8 in]
              n138 = in-place-cluster #3("USB IO.lvlib:USB IO.lvclass"=w316) -> (w300:T2)
            }
            n139 = Bundle By Name(cluster=T17 {"Module ID"=-1, "error"={"status"=FALSE, "code"=0, "source"=""}} ("read config (Reply Payload)"), "Module ID"=w303, "error"=w298) -> (w306:T17)
            n140 = Merge Errors(w312, w298) -> (w304:errorcluster)
            n141 = case "DQMH_FIRE_NOTIFIER" shown="True" w307 {
              tunnel: w308 -> [_ w319]
              tunnel: w306 -> [_ w318]
              frame False {
              }
              frame True {
                n142 = Send Notification(notification=w318, notifier=w319) -> ()  [unwired: 1 in, 2 out]
              }
            }
          }
          frame "init device" {
            n143 = property class="Mod Admin"(reference=w324) -> ("Accessors:Module ID"=w325:i32)  [unwired: 1 in, 2 out]
            n144 = Variant To Data(error in=w335, type=T9 {"Module ID"=-1, "Variant"=variant, "Wait Notifier"=refnum, "wait for reply"=FALSE} ("init device Argument"), Variant=w333) -> (data=w331:T9, error out=w334:errorcluster)
            n145 = Unbundle By Name(w331) -> ("Variant"=w320:variant, "Wait Notifier"=w330:refnum<notifier>, "wait for reply"=w329:bool)  [unwired: 1 out]
            n146 = in-place {
              in-place-border: [w337] -> w321
              in-place-border: w320 -> [w336]
              n147 = in-place-cluster #4(w323) -> ("USB IO.lvlib:USB IO.lvclass"=w339:refnum<class "USB IO.lvclass">)
              n148 = call-dynamic "init.vi"("Variant"=w336, "USB IO in"=w339) -> ("error out"=w337:errorcluster, "USB IO out"=w338:refnum<class "USB IO.lvclass">)  [unwired: 8 in]
              n149 = in-place-cluster #4("USB IO.lvlib:USB IO.lvclass"=w338) -> (w322:T2)
            }
            n150 = Bundle By Name(cluster=T18 {"Module ID"=-1, "error"={"status"=FALSE, "code"=0, "source"=""}} ("init device (Reply Payload)"), "Module ID"=w325, "error"=w321) -> (w328:T18)
            n151 = Merge Errors(w334, w321) -> (w326:errorcluster)
            n152 = case "DQMH_FIRE_NOTIFIER" shown="True" w329 {
              tunnel: w330 -> [_ w341]
              tunnel: w328 -> [_ w340]
              frame False {
              }
              frame True {
                n153 = Send Notification(notification=w340, notifier=w341) -> ()  [unwired: 1 in, 2 out]
              }
            }
          }
          frame "stop device" {
            n154 = property class="Mod Admin"(reference=w345) -> ("Accessors:Module ID"=w346:i32)  [unwired: 1 in, 2 out]
            n155 = Variant To Data(error in=w356, type=T10 {"Module ID"=-1, "Wait Notifier"=refnum, "wait for reply"=FALSE} ("stop device Argument"), Variant=w354) -> (data=w352:T10, error out=w355:errorcluster)
            n156 = in-place {
              in-place-border: [w357] -> w342
              n157 = in-place-cluster #5(w344) -> ("USB IO.lvlib:USB IO.lvclass"=w359:refnum<class "USB IO.lvclass">)
              n158 = call-dynamic "close.vi"("USB IO in"=w359) -> ("error out"=w357:errorcluster, "USB IO out"=w358:refnum<class "USB IO.lvclass">)  [unwired: 9 in]
              n159 = in-place-cluster #5("USB IO.lvlib:USB IO.lvclass"=w358) -> (w343:T2)
            }
            n160 = Unbundle By Name(w352) -> ("Wait Notifier"=w351:refnum<notifier>, "wait for reply"=w350:bool)  [unwired: 1 out]
            n161 = Bundle By Name(cluster=T19 {"Module ID"=-1, "error"={"status"=FALSE, "code"=0, "source"=""}} ("stop device (Reply Payload)"), "Module ID"=w346, "error"=w342) -> (w349:T19)
            n162 = Merge Errors(w355, w342) -> (w347:errorcluster)
            n163 = case "DQMH_FIRE_NOTIFIER" shown="True" w350 {
              tunnel: w351 -> [_ w361]
              tunnel: w349 -> [_ w360]
              frame False {
              }
              frame True {
                n164 = Send Notification(notification=w360, notifier=w361) -> ()  [unwired: 1 in, 2 out]
              }
            }
          }
          frame "analog read" {
            n165 = property class="Mod Admin"(reference=w367) -> ("Accessors:Module ID"=w368:i32)  [unwired: 1 in, 2 out]
            n166 = Variant To Data(error in=w378, type=T11 {"Module ID"=-1, "Line"="", "Wait Notifier"=refnum, "wait for reply"=FALSE} ("analog read Argument"), Variant=w376) -> (data=w374:T11, error out=w377:errorcluster)
            n167 = Unbundle By Name(w374) -> ("Line"=w364:string, "Wait Notifier"=w373:refnum<notifier>, "wait for reply"=w372:bool)  [unwired: 1 out]
            n168 = in-place {
              in-place-border: w364 -> [w381]
              in-place-border: [w380] -> w363
              in-place-border: [w379] -> w362
              n169 = in-place-cluster #6(w366) -> ("USB IO.lvlib:USB IO.lvclass"=w383:refnum<class "USB IO.lvclass">)
              n170 = call-dynamic "analog read.vi"("Line"=w381, "USB IO in"=w383) -> ("error out"=w379:errorcluster, "Voltage"=w380:dbl, "USB IO out"=w382:refnum<class "USB IO.lvclass">)  [unwired: 7 in]
              n171 = in-place-cluster #6("USB IO.lvlib:USB IO.lvclass"=w382) -> (w365:T2)
            }
            n172 = Bundle By Name(cluster=T20 {"Module ID"=-1, "Voltage"=0.0, "error"={"status"=FALSE, "code"=0, "source"=""}} ("analog read (Reply Payload)"), "Module ID"=w368, "Voltage"=w363, "error"=w362) -> (w371:T20)
            n173 = Merge Errors(w377, w362) -> (w369:errorcluster)
            n174 = case "DQMH_FIRE_NOTIFIER" shown="True" w372 {
              tunnel: w373 -> [_ w385]
              tunnel: w371 -> [_ w384]
              frame False {
              }
              frame True {
                n175 = Send Notification(notification=w384, notifier=w385) -> ()  [unwired: 1 in, 2 out]
              }
            }
          }
          frame "digital write" {
            n176 = property class="Mod Admin"(reference=w391) -> ("Accessors:Module ID"=w392:i32)  [unwired: 1 in, 2 out]
            n177 = Variant To Data(error in=w402, type=T12 {"Module ID"=-1, "Line"="", "On/Off"=FALSE, "Wait Notifier"=refnum, "wait for reply"=FALSE} ("digital write Argument"), Variant=w400) -> (data=w398:T12, error out=w401:errorcluster)
            n178 = Unbundle By Name(w398) -> ("Line"=w388:string, "On/Off"=w387:bool, "Wait Notifier"=w397:refnum<notifier>, "wait for reply"=w396:bool)  [unwired: 1 out]
            n179 = in-place {
              in-place-border: w388 -> [w405]
              in-place-border: w387 -> [w404]
              in-place-border: [w403] -> w386
              n180 = in-place-cluster #7(w390) -> ("USB IO.lvlib:USB IO.lvclass"=w406:refnum<class "USB IO.lvclass">)
              n181 = call-dynamic "digital write.vi"("On/Off"=w404, "Line"=w405, "USB IO in"=w406) -> ("error out"=w403:errorcluster, "USB IO out"=w407:refnum<class "USB IO.lvclass">)  [unwired: 7 in]
              n182 = in-place-cluster #7("USB IO.lvlib:USB IO.lvclass"=w407) -> (w389:T2)
            }
            n183 = Bundle By Name(cluster=T22 {"Module ID"=-1, "error"={"status"=FALSE, "code"=0, "source"=""}} ("digital write (Reply Payload)"), "Module ID"=w392, "error"=w386) -> (w395:T22)
            n184 = Merge Errors(w401, w386) -> (w393:errorcluster)
            n185 = case "DQMH_FIRE_NOTIFIER" shown="True" w396 {
              tunnel: w397 -> [_ w409]
              tunnel: w395 -> [_ w408]
              frame False {
              }
              frame True {
                n186 = Send Notification(notification=w408, notifier=w409) -> ()  [unwired: 1 in, 2 out]
              }
            }
          }
          frame "---Copy This Frame---" {
            # "Duplicate this frame when creating new messages.  Change this comment in the duplicated frame to describe this message."
            n187 = Merge Errors(w412) -> (w411:errorcluster)
          }
          frame "---Exit and Error Handling---" {
            # "Separator - the following cases handle errors and exit messages."
          }
          frame "Error" {
            # "#DQMH_CodeRecommended - If the module is running in standalone mode (External Launch = FALSE), this code will pop up an error dialog and call the 'Exit' message if an error occurs. Add more fine-grained error management here."
            # "Error - Check the error message data and respond accordingly. This message is sent by the \"Error Handler\" VIs at the end of each loop in this application."
            n188 = property on="Property Node" class="Mod Admin"(reference=w419) -> ("Accessors:External Launch"=w418:bool, "Accessors:Module ID"=w416:i32)  [unwired: 1 in, 2 out]
            n189 = Variant To Data(error in=w426, type=errorcluster {"status"=FALSE, "code"=0, "source"=""} ("error constant"), Variant=w420) -> (data=w415:errorcluster, error out=w424:errorcluster)
            n190 = local write "error out"(w415) -> ()
            n191 = call "Error Reported.vi"("Error"=w415, "Module ID"=w416) -> ()  [unwired: 9 in, 1 out]
            n192 = case shown="False" w418 {
              tunnel: [w431 _] -> w423
              tunnel: w417 -> [w429 _]
              tunnel: w415 -> [w430 _]
              frame False {
                n193 = disable-structure shown="Default" {
                  disable-tunnel: w430 -> [w432 _]
                  frame condition #0 (active) {
                    # "If the module is running standalone, then pop up an error dialog and call the \"Exit\" message."
                    n194 = call <vilib>:"Simple Error Handler.vi"("error in (no error)"=w432) -> ()  [unwired: 4 in, 5 out]
                  }
                  frame condition #1 {
                    # "To prevent the Simple Error Handler VI from being loaded (e.g. when deploying to a Real-Time target), add the Conditional Disable Symbol \"DQMH_Disable_SEH\" to your project and set it to TRUE."
                  }
                }
                n195 = call-poly <vilib>:"Delacor_lib_QMH_Enqueue Message (poly).vi"("Priority Message? (F)"=TRUE, "Message"="Exit", "Message Queue in"=w429) -> ("error out"=w431:errorcluster)  [unwired: 7 in, 1 out]
              }
              frame True {
                # "If the module was launched externally, calling the Error Reported broadcast VI is the only action performed by the \"Error\" message. The module's caller can then process the error appropriately."
              }
            }
            n196 = Merge Errors(w424, w423) -> (w422:errorcluster)
          }
          frame "Simulate MHL Error" {
            # "#DQMH_HowTo The 'Simulate MHL Error' button  illustrates how the MHL handles errors. This event is instructional in nature and can be removed."
            # "Simulate an error occurring at the MHL"
            n197 = property on="Property Node" class="Mod Admin"(reference=w438) -> ("Accessors:Module ID"=w439:i32)  [unwired: 1 in, 2 out]
            n198 = call "Module Name--constant.vi"("Module ID"=w439) -> ("Module Name"=w434:string)  [unwired: 10 in]
            n199 = Format Into String(format string="Simulated error originating at Message Handling Loop in %s", w434) -> (resulting string=w435:string)  [unwired: 2 in, 1 out]
            n200 = call <vilib>:"Error Cluster From Error Code.vi"("show call chain? (False)"=TRUE, "error message (\"\")"=w435, "error code (0)"=5001) -> ("error out"=w441:errorcluster)  [unwired: 6 in]
            n201 = Merge Errors(w443, w441) -> (w442:errorcluster)
          }
          frame "Exit" {
            w451 = 91  # 91: not all Exit messages will have an argument
            w452 = TRUE  # Stop the VI
            # "Release the message queue reference"
            # "#DQMH_CodeNeeded - Add any required cleanup code here."
            # "Exit - Exit the application."
            n202 = Variant To Data(error in=w460, type=T4 {"Module ID"=-1, "Origin"="", "Exit via Stop Module Req?"=FALSE, "Wait for Module to stop?"=FALSE} ("Stop Argument"), Variant=w450) -> (data=w447:T4, error out=w456:errorcluster)
            n203 = call <vilib>:"Clear Errors.vi"("error in (no error)"=w456, "specific error code to clear (0: all)"=w451) -> ("error out"=w459:errorcluster)  [unwired: 4 in, 1 out]
            n204 = property on="Property Node" class="Mod Admin"(reference=w445) -> ("Accessors:Module ID"=w444:i32)  [unwired: 1 in, 2 out]
            n205 = control-ref of="This VI"() -> (w446:refnum<vi>)
            n206 = call-dynamic "Delacor_lib_QMH_Release Message Queue.vi"("error in"=w459, "Message Queue"=w454) -> ("error out"=w458:errorcluster)  [unwired: 9 in]
            n207 = call "Handle Exit.vi"("Stop Argument"=w447, "Module Admin in"=w445, "VI reference"=w446) -> ("error out"=w457:errorcluster, "Wait for Stop?"=w448:bool)  [unwired: 7 in]
            n208 = Merge Errors(w458, w457) -> (w455:errorcluster)
            n209 = call "Error Reported.vi"("Error"=w455, "Module ID"=w444) -> ()  [unwired: 9 in, 1 out]
          }
          frame Default {
            # "'Default' case only runs if there is a message that isn't defined in any of the other cases.  Output a programming error."
            n210 = property on="Property Node" class="Mod Admin"(reference=w468) -> ("Accessors:Module ID"=w467:i32)  [unwired: 1 in, 2 out]
            n211 = call "Module Name--constant.vi"("Module ID"=w467) -> ("Module Name"=w461:string)  [unwired: 10 in]
            n212 = Format Into String(format string="The invalid message string \"%s\" was received in the Message Handling Loop for module \"%s\".", w462, w461) -> (resulting string=w464:string)  [unwired: 2 in, 1 out]
            n213 = call <vilib>:"Error Cluster From Error Code.vi"("show call chain? (False)"=TRUE, "error message (\"\")"=w464, "error code (0)"=1) -> ("error out"=w470:errorcluster)  [unwired: 6 in]
            n214 = Merge Errors(w471, w470) -> (w472:errorcluster)
          }
        }
        n215 = call-dynamic "Delacor_lib_QMH_Error Handler - Message Handling Loop.vi"("error in"=w228, "Message Queue in"=w219) -> ("dup error in"=w225:errorcluster)  [unwired: 8 in, 1 out]
      }
    }
    frame Error {
      n216 = call "Synchronize Caller Events.vi"("Module Admin"=w476) -> ("Module Admin out"=w475:refnum<class "Delacor_lib_QMH_Cloneable Module Admin.lvclass">)  [unwired: 9 in, 1 out]
      n217 = property on="Property Node" class="Mod Admin"(reference=w475) -> ("Accessors:Module ID"=w474:i32)  [unwired: 1 in, 2 out]
      n218 = call-dynamic "Delacor_lib_QMH_Release Message Queue.vi"("error in"=w482, "Message Queue"=w473) -> ("error out"=w481:errorcluster)  [unwired: 9 in]
      n219 = call "Module Name--constant.vi"("Module ID"=w474) -> ("Module Name"=w479:string)  [unwired: 10 in]
      n220 = Format Into String(format string="An error occurred during initialization. %s is no longer running.", w479) -> (resulting string=w477:string)  [unwired: 2 in, 1 out]
      n221 = call "Error Reported.vi"("Additional Information"=w477, "Error"=w481, "Module ID"=w474) -> ()  [unwired: 8 in, 1 out]
    }
  }
  n222 = Merge Errors(w17, w16) -> (w18:errorcluster)
  n223 = call "Close Module.vi"("error in"=w18, "Wait for stop?"=w2, "Module Admin in"=w4) -> ("error out"=w14:errorcluster, "External Launch"=w1:bool, "Module Admin out"=w3:refnum<class "Delacor_lib_QMH_Cloneable Module Admin.lvclass">)  [unwired: 6 in]
  n224 = Unregister For Events(event registration refnum=w9, error in=w14) -> (error out=w13:errorcluster)
  "error out" <- w13
  n225 = case "External Launch?" shown="True" w1 {
    tunnel: w13 -> [_ w483]
    frame False {
    }
    frame True {
      n226 = case shown="No Error" w483 {
        frame No Error {
          n227 = invoke class="VI" method="FP.Close"() -> ()  [unwired: 3 in, 3 out]
        }
        frame Error {
          n228 = disable-structure shown="Default" {
            frame condition #0 (active) {
              n229 = invoke class="VI" method="FP.Open"("Activate"=TRUE ("Activate?")) -> ()  [unwired: 4 in, 5 out]
            }
            frame condition #1 {
              # "Don't show panel on error if running inside a built EXE."
            }
          }
        }
      }
    }
  }
  n230 = local write "Module Admin"(w3) -> ()
